vi "Get Value by Name.vi"(8 "error in (no error)":errorcluster, 10 "Name":string, 11 "Values in":refnum<class "Values.lvclass">) -> (0 "error out":errorcluster, 2 "Value":variant, 3 "Values out":refnum<class "Values.lvclass">)   [LabVIEW 2020, in "HTTP Server.lvlib" / "Values.lvclass"]
uses:
  Values.lvclass
  Values.lvclass/Values.ctl
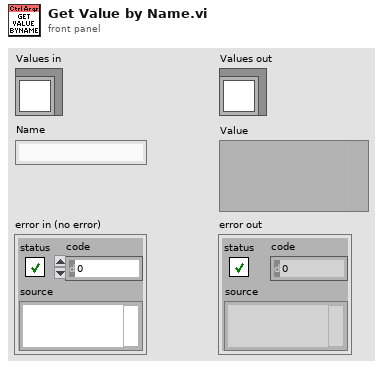
[diagram p1: front panel]
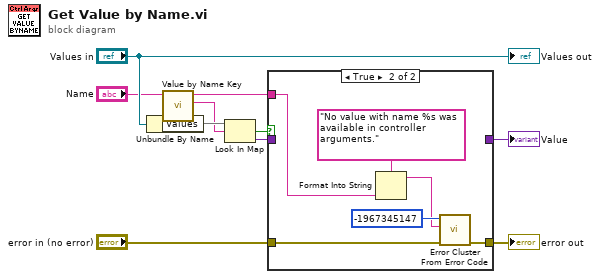
[diagram p0: block diagram]
diagram:
  n1 = Unbundle By Name("Values in") -> ("Values"=w10:map{string, variant})
  n2 = call "Value by Name Key.vi"("Value Name In"="Name") -> ("Value by Name Key"=w9:string, "Value Name"=w2:string)  [unwired: 9 in]
  n3 = Look In Map(map=w10, key=w9) -> (key not found?=w8:bool, value=w7:variant)  [unwired: 1 in]
  n4 = case shown="True" w8 {
    tunnel: w7 -> [w12 _]
    tunnel: "error in (no error)" -> [w11 w15]
    tunnel: [w11 w14] -> w1
    tunnel: w2 -> [_ w13]
    tunnel: [w12 _] -> w3
    frame False {
    }
    frame True {
      n5 = Format Into String(format string="No value with name %s was available in controller arguments.", w13) -> (resulting string=w17:string)  [unwired: 2 in, 1 out]
      n6 = call <vilib>:"Error Cluster From Error Code.vi"("error in (no error)"=w15, "error message (\"\")"=w17, "error code (0)"=-1967345147) -> ("error out"=w14:errorcluster)  [unwired: 6 in]
    }
  }
  "error out" <- w1
  "Value" <- w3
  "Values out" <- "Values in"
